vi "THIRD FPGA Speed Debug (RT).vi"() -> ()   [LabVIEW 2013]
uses:
  <vilib>/FPGAPlugInAG/sbRIO-9626/niLvFpga_Open_sbRIO-9626.vi
  <vilib>/rvi/interface/common/niFpgaWaitOnOcc.vi
  <vilib>/Utility/error.llb/Error Cluster From Error Code.vi
  <vilib>/rvi/errors/niLvFpgaAdjustHostInterfaceError.vi
  <vilib>/rvi/interface/nirviOpenFPGA/nirviOpenFPGA.xnode
  FPGA Bitfiles/SpeedFromFFT.lvbitx
  <vilib>/rvi/interface/nirviMethod/nirviMethod.xnode
  <vilib>/rvi/interface/nirviReadWriteControl/nirviReadWriteControl.xnode
  <vilib>/rvi/errors/niLvFpgaMergeErrorWithErrorCode.vi
  <vilib>/FPGAPlugInAG/sbRIO-9626/niLvFpga_ReadFifo_sbRIO-9626.vi
  <vilib>/ptbypt/NI_PtbyPt.lvlib
  NiFpgaLv.dll
panel:
  in  "PWM Duty":i32
  in  "PWM Period (ticks)":u32
  in  "tresh calc":bool
  in  "thresh":fxp<+/-,24,7>
  out "%diff speed":sgl
  in  "autostop":bool
  out "filt%diff":sgl
  in  "CommSegs":i32=8
  out "Waveform Graph":sgl[][](graph)
  in  "Hysteresis":fxp<+,10,5>
  out "actual time":dbl
  in  "Update Graph":bool
  in  "PresCtrl":fxp<+/-,20,5>
  in  "VoltCtrl":fxp<+/-,20,5>
  in  "PSenable":bool
  in  "Graph Refresh (s)":dbl
  # "Raw Current\nShift Ave Current\nThreshold\nRawP\nFilteredP\nAved P\nSpeed"
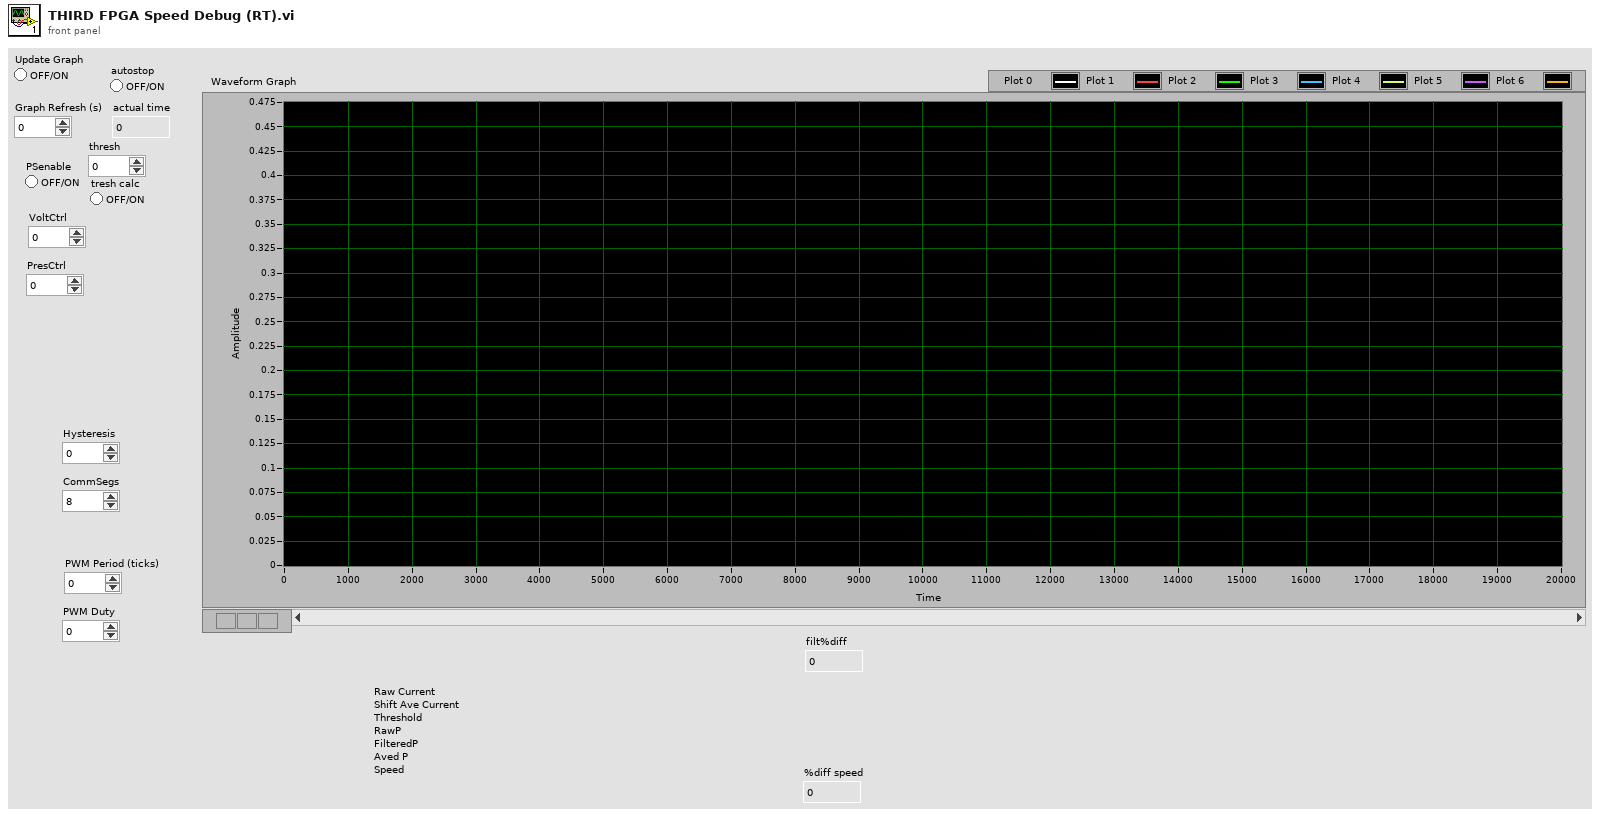
[diagram p1: front panel]
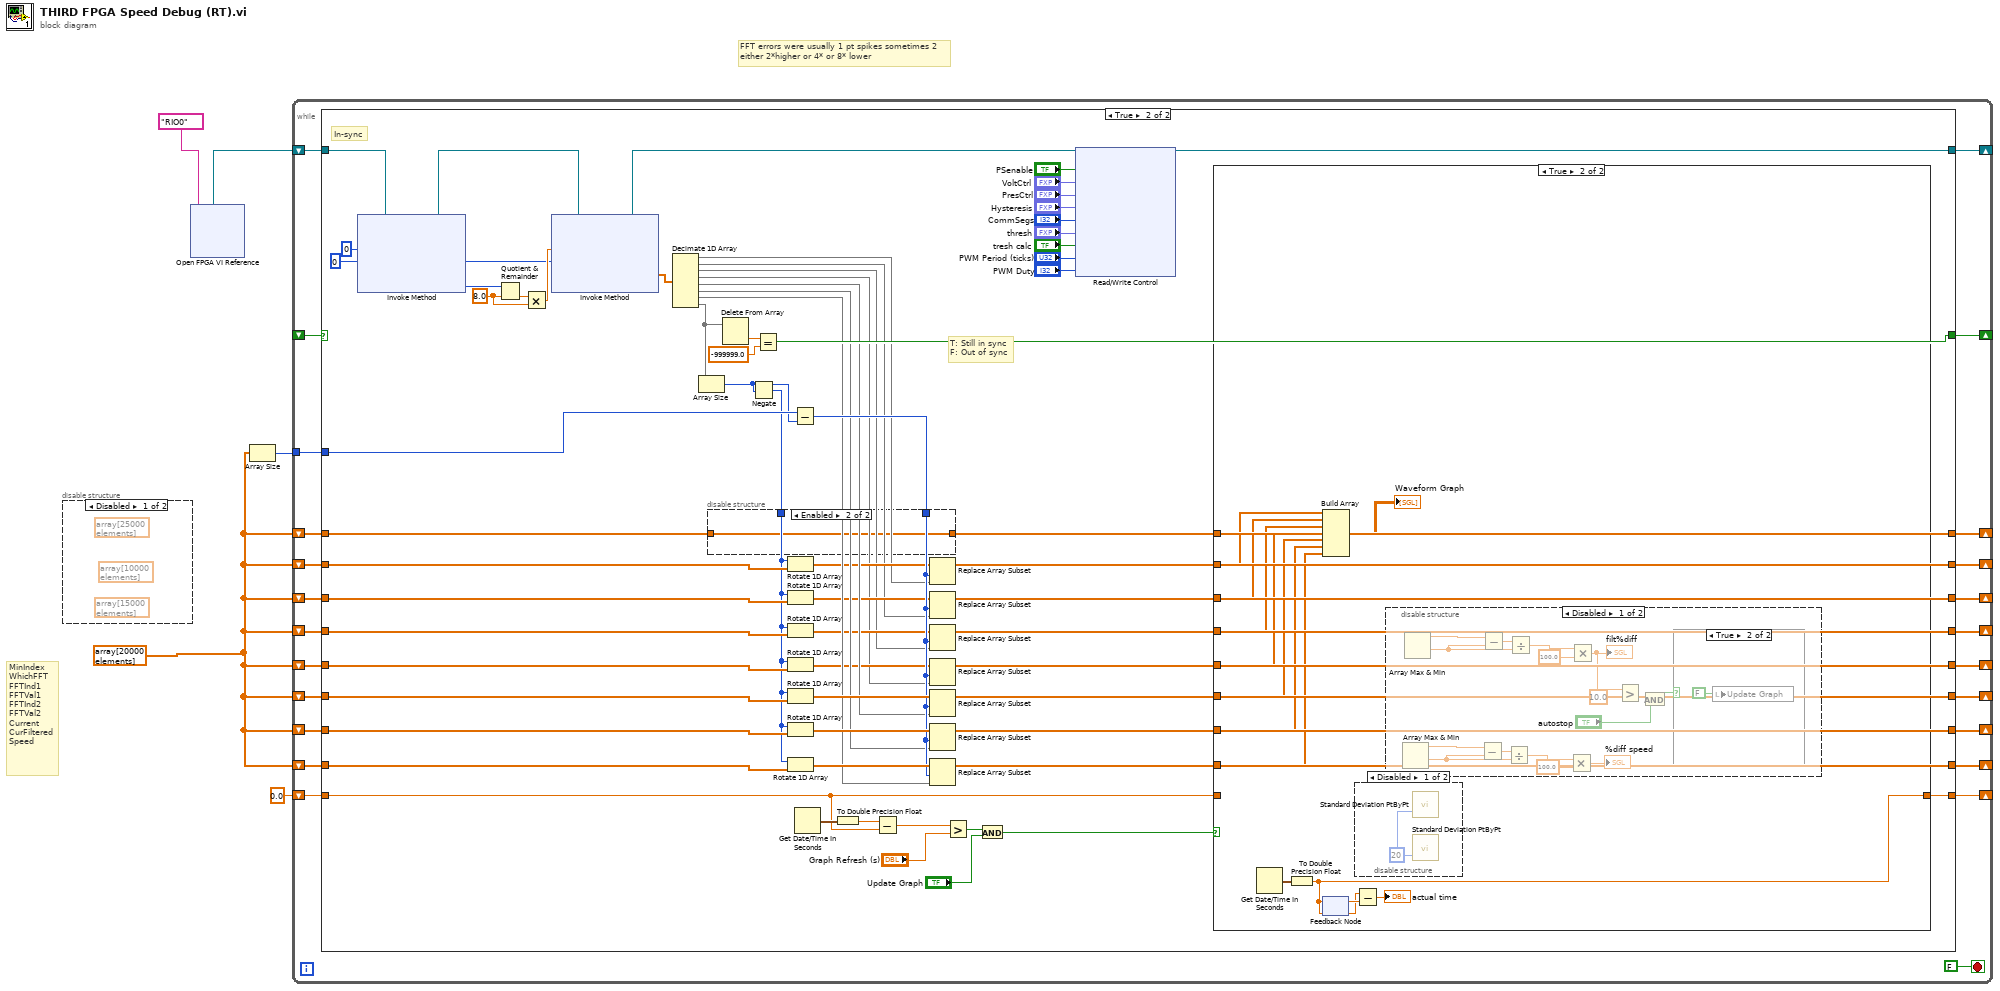
[diagram p0: block diagram]
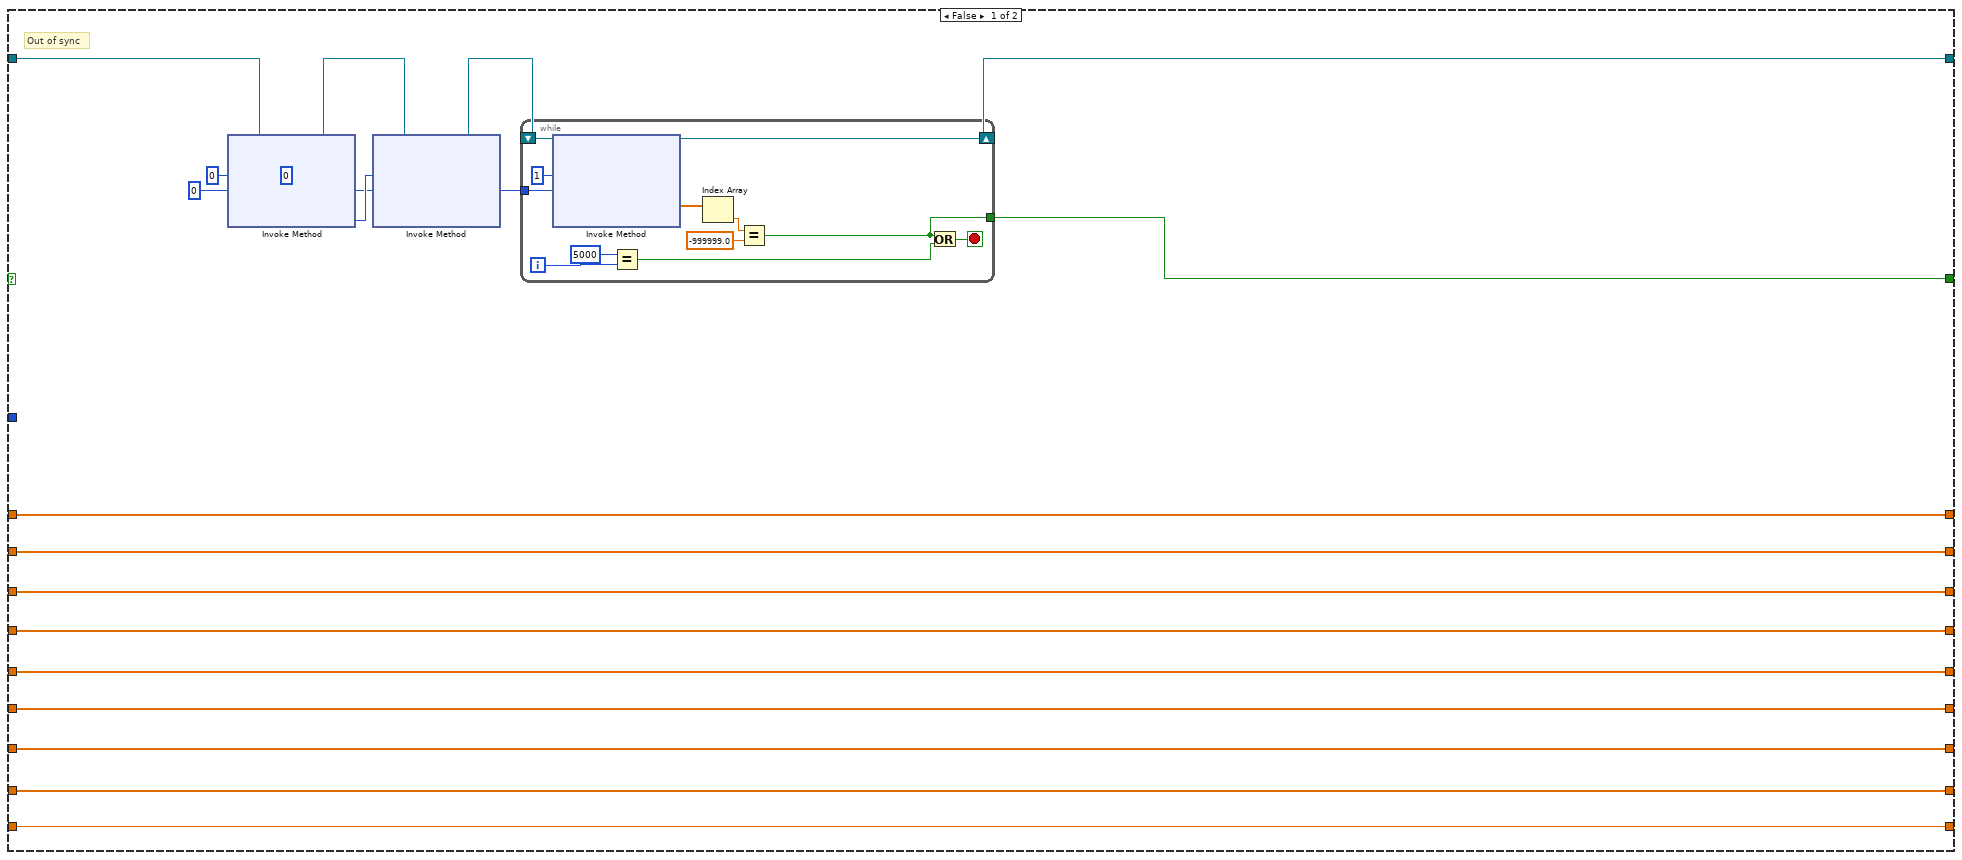
[diagram p3: hidden frame]
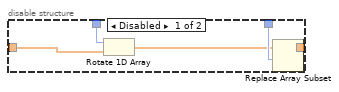
[diagram p4: hidden frame]
diagram:
  w1 = sgl[] array[20000 elements]
  # "FFT errors were usually 1 pt spikes sometimes 2\neither 2*higher or 4* or 8* lower"
  # "MinIndex\nWhichFFT\nFFTInd1\nFFTVal1\nFFTInd2\nFFTVal2\nCurrent\nCurFiltered\nSpeed"
  n1 = disable-structure shown="Disabled" {
    frame Disabled {
      (unwired) sgl[] array[10000 elements]
      (unwired) sgl[] array[25000 elements]
      (unwired) sgl[] array[15000 elements]
    }
    frame Enabled {
    }
  }
  n2 = xnode "Open FPGA VI Reference"("resource name"=tag "RIO0") -> ("FPGA VI Reference Out"=w5:refnum<k20>)  [unwired: 1 in, 1 out]
  n3 = Array Size(array=w1) -> (size(s)=w2:i32)
  n4 = while {
    shift-right: [w21] -> _
    shift-left: w5 -> [w28]
    shift-right: [w26] -> _
    shift-left: _ -> [w29]
    shift-right: [w24] -> _
    shift-left: w1 -> [w25]
    shift-right: [w23] -> _
    shift-left: 0.0 -> [w22]
    shift-right: [w20] -> _
    shift-left: w1 -> [w18]
    shift-right: [w19] -> _
    shift-left: w1 -> [w17]
    tunnel: w2 -> [w16]
    shift-right: [w11] -> _
    shift-left: w1 -> [w10]
    shift-right: [w12] -> _
    shift-left: w1 -> [w9]
    shift-right: [w13] -> _
    shift-left: w1 -> [w8]
    shift-right: [w14] -> _
    shift-left: w1 -> [w7]
    shift-right: [w15] -> _
    shift-left: w1 -> [w6]
    stop <- FALSE stop-if-true
    n5 = case shown="True" w29 {
      tunnel: w28 -> [w45 w119]
      tunnel: [w41 w121] -> w26
      tunnel: w25 -> [w40 w120]
      tunnel: [w40 w88] -> w24
      tunnel: [w39 w90] -> w23
      tunnel: w22 -> [w39 w89]
      tunnel: [w37 w98] -> w21
      tunnel: [w36 w87] -> w20
      tunnel: [w35 w86] -> w19
      tunnel: w18 -> [w36 w107]
      tunnel: w17 -> [w35 w106]
      tunnel: w16 -> [_ w101]
      tunnel: [w34 w85] -> w15
      tunnel: [w33 w84] -> w14
      tunnel: [w32 w83] -> w13
      tunnel: [w31 w82] -> w12
      tunnel: [w30 w81] -> w11
      tunnel: w10 -> [w30 w96]
      tunnel: w9 -> [w31 w95]
      tunnel: w8 -> [w32 w94]
      tunnel: w7 -> [w33 w93]
      tunnel: w6 -> [w34 w92]
      frame False {
        w38 = 0 ("Timeout (ms)")
        (unwired) u32 0 ("Number of Elements")
        # "Out of sync"
        n6 = xnode "Invoke Method"("FPGA VI Reference In"=w45, "Number of Elements"=u32 0, "Timeout (ms)"=w38) -> ("FPGA VI Reference Out"=w44:refnum<k20>, "Elements Remaining"=w43:u32)  [unwired: 1 in, 2 out]
        n7 = xnode "Invoke Method"("FPGA VI Reference In"=w44, "Number of Elements"=w43, "Timeout (ms)"=w38) -> ("FPGA VI Reference Out"=w42:refnum<k20>)  [unwired: 1 in, 3 out]
        n8 = while {
          shift-right: [w49] -> w37
          shift-left: w42 -> [w58]
          tunnel: [w48] -> w41
          tunnel: w38 -> [w47]
          i -> [w53]
          stop <- w50 stop-if-true
          n9 = xnode "Invoke Method"("FPGA VI Reference In"=w58, "Number of Elements"=u32 1, "Timeout (ms)"=w47) -> ("FPGA VI Reference Out"=w49:refnum<k20>, "Data"=w56:sgl[])  [unwired: 1 in, 2 out]
          n10 = Equal?(x=5000, y=w53) -> (x = y?=w51:bool)
          n11 = Index Array(array=w56) -> (element=w55:sgl)  [unwired: 1 in]
          n12 = Equal?(x=w55, y=sgl -999999.0) -> (x = y?=w48:bool)
          n13 = Or(x=w48, y=w51) -> (x .or. y?=w50:bool)
        }
      }
      frame True {
        w111 = 0 ("Timeout (ms)")
        w124 = 8.0 ("y")
        # "T: Still in sync\nF: Out of sync"
        # "In-sync"
        n14 = xnode "Invoke Method"("FPGA VI Reference In"=w119, "Number of Elements"=u32 0, "Timeout (ms)"=w111) -> ("FPGA VI Reference Out"=w116:refnum<k20>, "Elements Remaining"=w118:u32)  [unwired: 1 in, 2 out]
        n15 = Quotient & Remainder(x=w118, y=w124) -> (floor(x/y)=w125:dbl)  [unwired: 1 out]
        n16 = Multiply(x=w125, y=w124) -> (x*y=w117:dbl)
        n17 = xnode "Invoke Method"("FPGA VI Reference In"=w116, "Number of Elements"=w117, "Timeout (ms)"=w111) -> ("FPGA VI Reference Out"=w102:refnum<k20>, "Data"=w115:sgl[])  [unwired: 1 in, 2 out]
        n18 = Decimate 1D Array(w115) -> (w63:sgl[], w64:sgl[], w65:sgl[], w66:sgl[], w73:sgl[], w72:sgl[], w71:sgl[], w77:sgl[])
        n19 = Array Size(array=w77) -> (size(s)=w100:i32)
        n20 = Delete From Array(array=w77) -> (deleted portion=w122:sgl)  [unwired: 2 in, 1 out]
        n21 = Negate(x=w100) -> (-x=w74:i32)
        n22 = Equal?(x=w122, y=sgl -999999.0) -> (x = y?=w121:bool)
        n23 = Rotate 1D Array(1:w107, 2:w74) -> (0:w70:sgl[])
        n24 = Rotate 1D Array(1:w106, 2:w74) -> (0:w69:sgl[])
        n25 = Rotate 1D Array(1:w92, 2:w74) -> (0:w68:sgl[])
        n26 = Rotate 1D Array(1:w93, 2:w74) -> (0:w67:sgl[])
        n27 = Rotate 1D Array(1:w94, 2:w74) -> (0:w78:sgl[])
        n28 = Rotate 1D Array(1:w95, 2:w74) -> (0:w79:sgl[])
        n29 = Rotate 1D Array(1:w96, 2:w74) -> (0:w76:sgl[])
        n30 = Subtract(x=w101, y=w100) -> (x-y=w75:i32)
        n31 = disable-structure shown="Enabled" {
          disable-tunnel: w120 -> [w130 w131]
          disable-tunnel: [w129 w131] -> w88
          disable-tunnel: w75 -> [w128 _]
          disable-tunnel: w74 -> [w127 _]
          frame Disabled {
            n32 = Rotate 1D Array(1:w130, 2:w127) -> (0:w126:sgl[])
            n33 = Replace Array Subset(array=w126, index=w128) -> (w129:sgl[])  [unwired: 1 in]
          }
          frame Enabled {
          }
        }
        n34 = Get Date/Time In Seconds() -> (seconds since 1Jan1904=w114:timestamp)
        n35 = To Double Precision Float(number=w114) -> (double precision float=w99:dbl)
        n36 = Subtract(x=w99, y=w89) -> (x-y=w113:dbl)
        n37 = Replace Array Subset(array=w70, new element=w63, index=w75) -> (w87:sgl[])
        n38 = Replace Array Subset(array=w69, new element=w64, index=w75) -> (w86:sgl[])
        n39 = Replace Array Subset(array=w68, new element=w65, index=w75) -> (w85:sgl[])
        n40 = Replace Array Subset(array=w67, new element=w66, index=w75) -> (w84:sgl[])
        n41 = Replace Array Subset(array=w78, new element=w73, index=w75) -> (w83:sgl[])
        n42 = Replace Array Subset(array=w79, new element=w72, index=w75) -> (w82:sgl[])
        n43 = Replace Array Subset(array=w76, new element=w71, index=w75) -> (w81:sgl[])
        n44 = Greater?(x=w113, y="Graph Refresh (s)") -> (0:w109:bool)
        n45 = And(x=w109, y="Update Graph") -> (x .and. y?=w91:bool)
        n46 = xnode "Read/Write Control"("FPGA VI Reference In"=w102, "PSenable"="PSenable", "VoltCtrl"="VoltCtrl", "PresCtrl"="PresCtrl", "Hysteresis"="Hysteresis", "CommSegs"="CommSegs", "thresh"="thresh", "tresh calc"="tresh calc", "PWM Period (ticks)"="PWM Period (ticks)", "PWM Duty"="PWM Duty") -> ("FPGA VI Reference Out"=w98:refnum<k20>)  [unwired: 1 in, 1 out]
        n47 = case shown="True" w91 {
          tunnel: [w132 w141] -> w90
          tunnel: w89 -> [w132 _]
          tunnel: w88 -> [_ _]
          tunnel: w87 -> [_ w133]
          tunnel: w86 -> [_ w134]
          tunnel: w85 -> [_ w135]
          tunnel: w84 -> [_ w136]
          tunnel: w83 -> [_ w138]
          tunnel: w82 -> [_ w139]
          tunnel: w81 -> [_ w137]
          frame False {
          }
          frame True {
            n48 = Get Date/Time In Seconds() -> (seconds since 1Jan1904=w144:timestamp)
            n49 = To Double Precision Float(number=w144) -> (double precision float=w141:dbl)
            n50 = feedback #1(w141) -> (w142:dbl)
            n51 = feedback-in #1(w141) -> ()
            n52 = Build Array(w133, w134, w135, w136, w138, w139, w137) -> (→"Waveform Graph":sgl[][])
            n53 = disable-structure shown="Disabled" {
              frame Disabled {
                w162 = 20 ("sample length")
                n54 = call <vilib>:"Standard Deviation PtByPt.vi"("sample length"=w162) -> ()  [unwired: 2 in, 3 out]
                n55 = call <vilib>:"Standard Deviation PtByPt.vi"("sample length"=w162) -> ()  [unwired: 2 in, 3 out]
              }
              frame Enabled {
              }
            }
            n56 = Subtract(x=w141, y=w142) -> (x-y=→"actual time":dbl)
            n57 = disable-structure shown="Disabled" {
              frame Disabled {
                n58 = Array Max & Min() -> (max value=w145:dbl, min value=w147:dbl)  [unwired: 1 in, 2 out]
                n59 = Array Max & Min() -> (max value=w160:dbl, min value=w158:dbl)  [unwired: 1 in, 2 out]
                n60 = Subtract(x=w145, y=w147) -> (x-y=w146:dbl)
                n61 = Subtract(x=w160, y=w158) -> (x-y=w159:dbl)
                n62 = Divide(x=w146, y=w147) -> (x/y=w148:dbl)
                n63 = Divide(x=w159, y=w158) -> (x/y=w157:dbl)
                n64 = Multiply(x=w148, y=sgl 100.0) -> (x*y=→"%diff speed":dbl)
                n65 = Multiply(x=w157, y=sgl 100.0) -> (x*y=w155:dbl)
                "filt%diff" <- w155
                n66 = Greater?(x=w155, y=sgl 10.0) -> (0:w153:bool)
                n67 = And(x=w153, y="autostop") -> (x .and. y?=w152:bool)
                n68 = case shown="True" w152 {
                  frame False {
                  }
                  frame True {
                    n69 = local write "Update Graph"(FALSE ("Update Graph")) -> ()
                  }
                }
              }
              frame Enabled {
              }
            }
          }
        }
      }
    }
  }
